vi "Puzzle 14-2.vi"() -> ()   [LabVIEW 2022 SP3]
panel:
  in  "delimited string":string="...#.O.#.#.O.O....#...O....#..#........OO.O#...O..O#O#.......O.O....O.....#...OO#.O....OOO..OO#..#..\n.##.....#.OOO.OO#...O.......O#..O.##OO.O.......O##....O....#O..O..#.#....#OO..#...O.O#.#...#....#O.O\nO...##.O.O.O.O..#.#.....#O....#..#O..O...O..OO..O...##.......OO#..OOO..#O..#.O#.O......#..#O..O..O.O\n..OO....OOO....O.O..OOO.....O........#...O.O.O.O..O#.O...O..#.#O........O.....#O...##....#...#.#....\n##.O.O#..O..##O.....O.#.....O.O#O.O..#...#...OO.##OOO...OO#...O...O........O.#.O.........#O.#...#.#.\n.#.O.O.....#..O###..O#.#..O....O.O....#...##.O..O.OOO..O.O..O#.O..O....#.#.O..#..##O...O....#O#.....\n.......O...##..O..O##..##...O....###.O.#.#.O......O...O.O......#O.....#..O..O#..##O.O#O##O....O#....\n.#O..#....##.##..O#..#..#..O........OO....#..##.O.#.O.O..OO.O.O#..#O##O......OO...O...OO...#....OO..\n#.....O#......O#.....#..O...#O..OO..OO.#O...O...O.........O...#O...O.....#.....#...#.....O##.O.....O\nOO.O..O...O......#.O......#O....#..#.#...O.O....O.#.O#...O........O......#.#O#.O...O.........#O....O\nO.O..O..#......O.O.OO...OO..##.....OO.....#.O...O.#.#...OO..OO.O.........#O..#.O...O#.#..O..OO.##O..\n..#.......O....#...#....##..O.O......O....O#.O..O..#.#.O#O.O.#...#.##.....O...O.O...O.#...O...O.#...\n.O...#..O.....O.O.....OO.O.O.......O..O..........#...O..O..O......O....#OOO...O#O...#.O#........O...\n.OO#....#.....O...#.###..#..O..O.....#O..#..OO...OOO#.O#..O#O........#..#.O..OOO#O#..O..OO........#.\n..O.....#..#..O.............#..O.O..O#.......#.O.........O.#..OO.O..#..##..O.O#O....OO.O.O.O.....O#.\n........#O..O#OO...#.##O.O....O...O..........##.#O..O......O..O.#...#O.O.OO...#.#OOO.#...O#....#.O.#\n.....O.O...#OO#.OO#......#..O.O..#.OO.......#...#.O.O#.O.#O.O#..#O##..OO...#......#.O....#.....O.#O.\n.O#OOOO...#.#..........O#.#.#.#.O....O..O...O...OOO.O.O.O..OO..O..O#.#...#....#...#O#.OO.O..#.O#....\nOO#OO..#.O.#....#..#.#..#O#.O#O#.#..O.O....#..O...OO..O..#........#.O...O#.#.....#....O.....#.O.....\n.O.....#...OO...#..O..#..O..O##..OO...O....#.O.#............###.O.#..O..O.........O..#.O..O.#OO.#...\n.##O.#.O.#....O..O..#..O.#.O..##O..O......OO...#...O..OO#....O..O#O.##.OO#...O#...#.......O.O#.#OO..\n.OO#O#...O..##.O......O..O.O....O...OOO.O..#...O#.#.O.OOO..#...#.##..OO..................OOOOO...###\n.#..##...####.O#...O........O...#O..O..O....O##O..O..OO..#.....#...O.....OO......OOO.#..O.##OO##...#\n....O#........O##.O...O#..#.O#O...O...O.O........#..#.#.O......O..#.....#.O..#.#..#..#O....O##...#..\n.O..OO.O##..O...O.OO....O.OOO..#O#.O##......O.O#....O#O.O......#.O..#O..#O.........#..OO....#.OO..O.\n.#OO..#OO.###........#...#..#.O..#O.O#O...O.#.....O...#......O.......#.O.#.##.O..#O.O###OOOO...#..O.\n##...OOO.#..........O#...O#.....OO...O#..OO.OO.#.OOO..OO....O..OOO...##O...O.........##O...#.#O.....\n.#....O.....#OO.O.OO..O......#.OO..#O...O..##O.#O....#O.OO..#O.OO...O..O.#..##...O......#O##OO.#.O..\n.#..O....O....#......#.O.##...OO.O.O...O.OO.O....#...#..O....O#O..#...#.#..#...OO......OOO...O..#...\n#.#OO.#....O.#.OO....#........O.O.##...O.#.................OOOO....O..#......O..#.#...O....#.O#OO.#O\n....O.O.......##..O.........OO#O..O.O#.#.#.O....#..OO.O..O#O....O..O.O......O.O.#..O.......O.O..O.O#\n...........#OO...O....#.O.#..#O.O#.....O..O.....O#.....OO.#O...#O.#O.#.....OO.O.O....OO......O#O.O..\nOOOO.OO..O....O.O...O..#.........O#.##OOO#.O..O.O.O......O..#..O..#..#.O..O....O#O.#OO..O.O...O#.##.\n##.O.#O.#OO#..........OO#.OO.#..#.#......#.OO...#.O.O.......O##....O..O..#.#.#O....O..##.#OO.O..O..O\n#O...OO..#.#....##.O#.#...##OO#........O#.O..O#.........O.O.#....O.#.O.......O..OOO......O#O.###.O..\n....O#....#..O...#.#.....O.O#O..#O....O...O.OO#...O..O#.##.O.....O...#..#.O.....O...O#..O.#...#.#O..\nO.OO......#..O...O.O....#...OO..O#.O..OO..#.##.....#....O.O#O#.O....O..#..OOO..O....O.O..#..O.O..O..\n.#..#..##O..O.....O#.#.O.O..O..OO..O.O..OO.##.O...O..O#........O.............#.OO..#......O..#O#OOO.\n.#..##...O.#..OO...O..#..#O#..#..##.O#.#.....#....O.O..O.........#.###...#.O##..O...#.O.OO..........\n........#O.......O...O#.#....#.O#....#..O.....OO........O...#.........##.....O...O#.O...O.O..#OO.O.#\n.#..#.O##..##.O#.#.......OO...OO#...#O#............#.#...#...O...#.O..#O.#.O.........O..OO.O...O.#..\n#.O#OO...OO.O.#...##........#....O.#.O.....##.#.O.O.O.#..O#...O..#......#..O...###O..OO..##..OO.#OOO\n.OO...#O....O##.O...O.#....O...#O.......O.....OO.O...O..#...OO.OO.O#...O##.....O..#.#...#OO......O..\n..O..#...O...##..O...O..OO.O.O.O.....#.....O.....O..#OOO.....OOOO#.#.O..O..#........O.#O#.#O..O.##..\n.....##.....O.....O#...##.OOO....O.O..O.#.#O........OO.....#...##...#.#......#....OO.O.....#O....#.#\n..O.OO#....O..O.#O.#OO#..#.O.##.#..#.OO##....O#...#..O.#..#...#.#....OOOO.#...OOOO..O.........##O.O.\nO.O.#......O#...O..#.......#O.O..OOOO..#....#.#.OO.O..#O......#.#....#...#..O....#O.OO..O.......#.#.\n...O.O....O#......#.O.O....O#.#..#O.#.....#...#...#.O#.........O.OO..O###...O....O.#.O.#.....##..O..\n.#.OO...O#O.....O#....O......OO...OO.OOOOOO##....#..#..#O.#.OO....O#..OO.#O........O#..O.O#.#.......\n#OO#.#.....O#OOO#...O.........#......O#.......O.....O#.#O...O........#....O...O.....#.......##.OOO#.\n..#.O##..#OO..#....#O....#....#..........#O...#...O.#.O.O###O..O..#...#.OO....##..O.O.O.....O..O....\n....OOO#.#......#..O.O......##O.#.O.#.O.OO....#..O.......#.....#O.O...##O###.##.##..#.O.#.O#..#..O#.\n......O#OO......#.#..#.O#OO#O..O#O.O##.......O...O........O......O#.....#..#....#...#.#..O...O##.#O.\n#..OO..O.O.....#O.O.#.#......O......O.#....O.#OO.........#.O.O#..#..#.O..O.#..#...#...O.#..........O\n..O#OOO#.#.....O.....O..##.#..OOO.O..#..O#...##O..OO...#....#..#...#...OO.....##OO#.OO...#.O....#.#.\n#.#O.............#....O#.....O.....O.##O.....#.#.#.....O....O...O...##..O...#........#O..##.#.....##\n.O.....O...#O.#.O#..O#........#.##...O##O..........O##.O......O..#....##....###......O##..##O..#.O#.\n.#...#..#..O.O.............#....O.OO.....OO#O.....OO..OOO#O.O.O.O...#...#.........OO..O#.O...#.##..#\n..O...#O#.......#OO..........OO#..#.....OO#...#OO.O#....OO....O..O..#....#OO......O#O...#......O..O.\nO.......O..O..#O.....O#O.........O##.O#.#.O.O....##....O.#....O....OOO..#O#...#...O.O#.O.....O.O#.O.\nO.#O....O..##....O.........##.OO###....O...O...O..O#O#...#O.O.O....#..O..#..#.O.......###..#....#..O\n.........O..#O...O..OO.....#...O..#O#.....O....#O#....##...#.OOOO.O..O#...O..O.O#.#..O.O..#..#.OO...\n...#.....#..OO.O.#.#.O.....O#...#..O...O..O..#...O..O.O..#...#.###..#..##O.#.#O.......O..##O.O.O#...\n.##O......O....#....O....#O..#.....#.O..O.O.O..#.#O.....O#.O...#.#O.#...#.........O....O....OO..O...\n.OO.O.O.O#O..O##.O...OO.....O..O....O....#..#...O.O...O....O.#.O......#O.#.O#O..O...O.O.#.O..O.#....\nO#..#.#..#..#...#.O...O.###.##.OO.O.#.OOO..O..#O.#.O...OO...O.OOO....#.....#OO.O##.O.#.#O...#.#.....\n.#.....#.........O.#.........#...OO..O.#.O...O##O...#..O.O.OO#....###.OO.....#..........#.#OO...O.O.\n........OO..O.O.#..O.#.......#.#O.OOO...OO.O............O#O#...O...#.O.....#...........O...#..OO.O#O\n..#.#.#...O....#O.......#...#...O###.O.....O.O.OO....#O...OO.O.O........O.O.#O.O....OO.....OO.....#.\n#..OOO#......O.#.O#...#..#..O..O.O.O.#...O#OOO.#...O.#.OO.#O..#....#..#O....O.#.O...O...O#OO...#....\n.....#.....##...O....#..O..O.....O#OO.#O#.....O...O.##.#........O..O........#.#......##......#..#..O\nO..O....O.##..#.#O##.#.....OO....O.##O......#...#..OO.O.....#...#........O..O#O##.O.......#..##O..##\n#.....#O....O...#OOO#..O#.O.....O..OO.#..#.#.O#..O..O#.O###....O......O.#.O..#O.....#.......##O.O..O\nO.O.#..#....O....O.......#.O..O#O#.O..........#O.....#OO.O...#.OO.....#...O....OO....#...O....O.#..O\n..#...OO....OO......O....#..#..........##..##..#.....##...#..#O.....#OO......#........O.....O..O...#\n.OO#...O#.O....#.........OO#...O#..O.#..O.O.O.#O......##.O.......O...O...###.O......O....O...#.OO#..\n..O..O#O.#..O.#O...OOO#O.#.O....O.#......O....#....###....OO......O...#...OO.#....O........O#..#..OO\n#..OO..O......#...##..O#.O........O.O...##.#O...O...#O#.O.O....#.............#.O#.#..O..#..OO#.....#\n#..........O...O##.O#..O..OO..O.....#O.#.O......#......O.O....##.O#OO..O.O..O.O.O..#..O....O..#....O\n.O.O...O.#..O.O....#.#.O.O.##.##..O..#OOOO.###...#O...#...O.....O...#.##.OO..O.#..#.O.#.......O....#\n#....#....OOOOOOO.#...OO....##O.#..#......O..#..........O......##..O..###..#.O....O.......OO......#.\n.O.O..##.O.#O.#...#....O..O.....#..##......O.......O..O#.O##.#........O..#.O.#.O.O..##..###..##.#...\n..OOO..O##..OOOO.O.....OO##..O..O.#....#.....OO......O.OOO#...#O.OO...O.O......O#..O.##....###...#.O\n....O...O.O....#..O#.O.....O.O.#.......O##...O#..OO.O.O##...#.....O#.###....O....#O.........OO..O.O.\nO#.O......##..#.#..............#......#.#.OO#......##O#OO..OOO..##.O##....#..O...#......##O.O##...OO\n...#OO....OO...O#.#..##....OO.#..#O......O#....#.O.....O.#O..OO.#..OO...O#.O#....O.#.OO.O.O#..O.....\n#..O.OO#O...O..O..........#..#.#..#..#O.....#O#..O....#..O...O.#.#O#.#OO.....OOO.#..#.........O...O#\n....O......#..........O...#.....OOOO........#.#OO.O............O...#....O........#....#....#........\n...O.......###...O.O...#O.##O.OOO.........O.###.O.......O....O.O...O.#.....#..#O..#..OO..O.O...O....\nO.O#....##.O.O.....O....#............OO.#O...O..#...##.#.#O#O.#.....O......O....#.OO#.O#....#.....O.\n..O####.O.........O...........OO..OO.#.....O.......#..O#.O....O#...##.......#.#....O..O..O#..##.....\n.#..#......O.##.O.OOO.O.OO....O.......#......#.O...OOOO...O..#..#.O.#......O...O#.#.O.#.O....O....O.\n##....O.O..O..O.#...O##.......O....#...#OOO.O..##.....#....O.......#O..#.#O..O.#.......O..#.O.O#.O##\n...O....O#O.#...#......#..O.O.O.O...O.....O..O.#..#.....O#...OO...#.O.O....#..OOO...#.....OO.OO..O..\nO##.O.##.O#OO...OO...OO..O....OO#O.#O..O.O....OO..........O..#.O.#O#.......O.O..#O#....#..#...#O..#.\n.#.#..........#.......#..OO#....O.#.#.O.....OO.#.O..#.#.O....#..O....#..#..O.#O#O.....#.O.O.#O.O.#O.\n.O.#....##O...#..OOO.#......#...#.O.......OO....#.......#..#.OOO........OO..O..###O##..O.....O##....\nOO##..O#....O.##.......O...#........O.O...#O#.#.OOO....#......#.#O.O.O..O..O...#.#.O.O.OOO.O#O......\n#O...#....OOO.O...#O....O...O..........O..#..O#.O..#O.....#......#.#..#.OO..#....#O#....O...O....##.\n.OOOO......##.#O.#O...#......O..#..O..#.O...O.OO...............#O...O..##..#.#....O...O..O.##..O.O.."
  in  "Numeric":i32=1000000000
  out "sum":i32
  out "unsigned byte array 2":u8[][](array[numeric])
  out "unsigned byte array":u8[][](array[numeric])
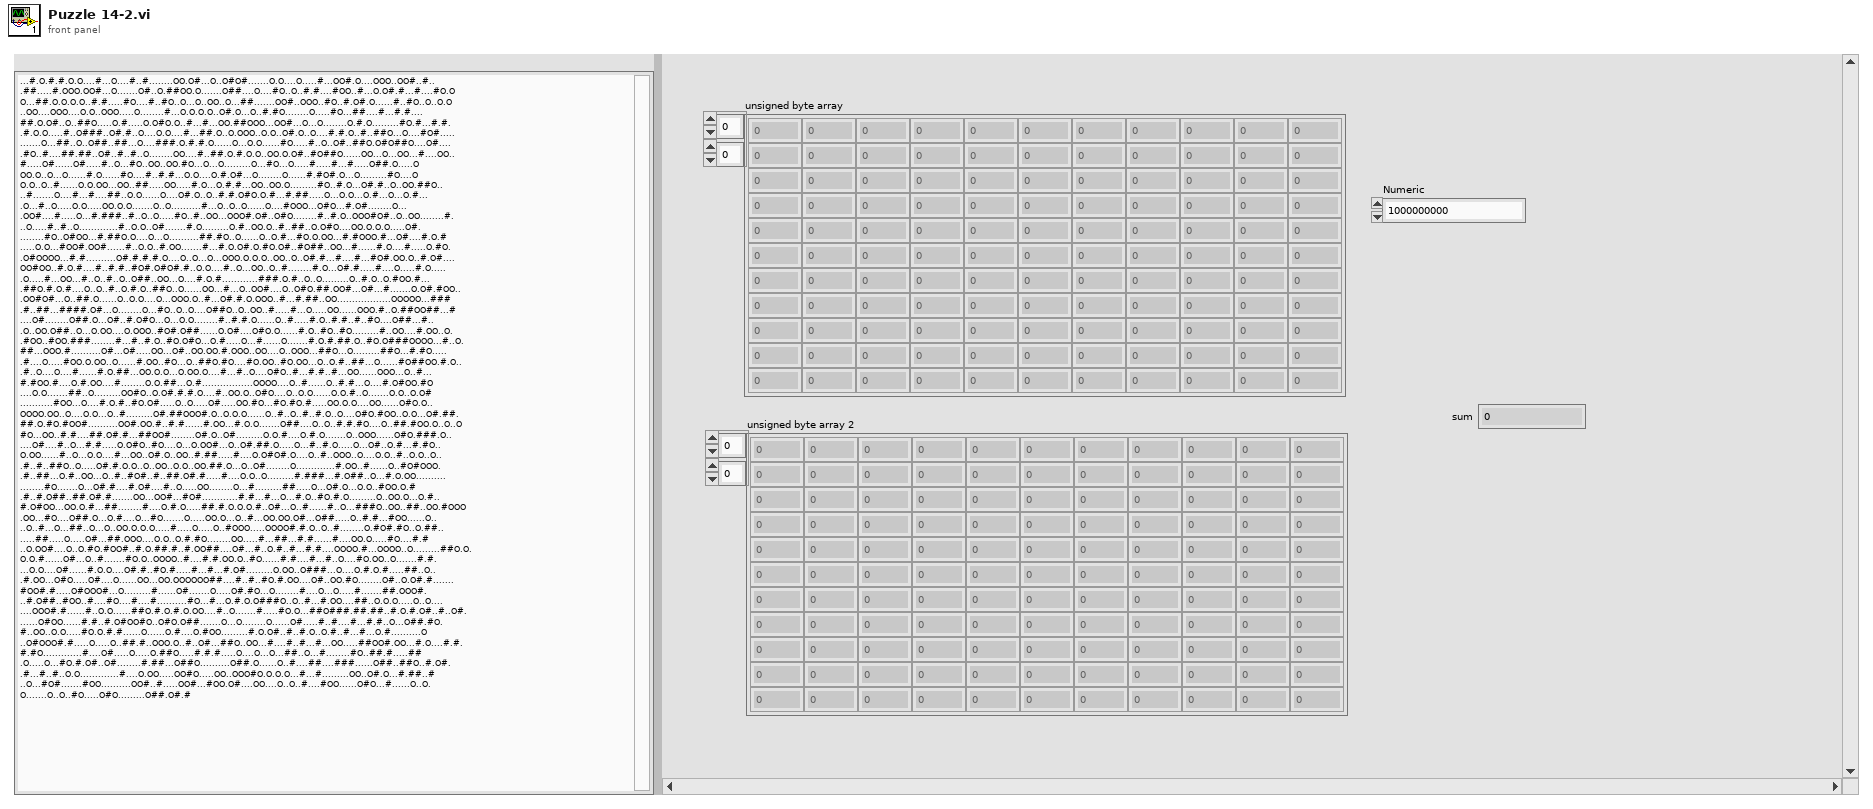
[diagram p1: front panel]
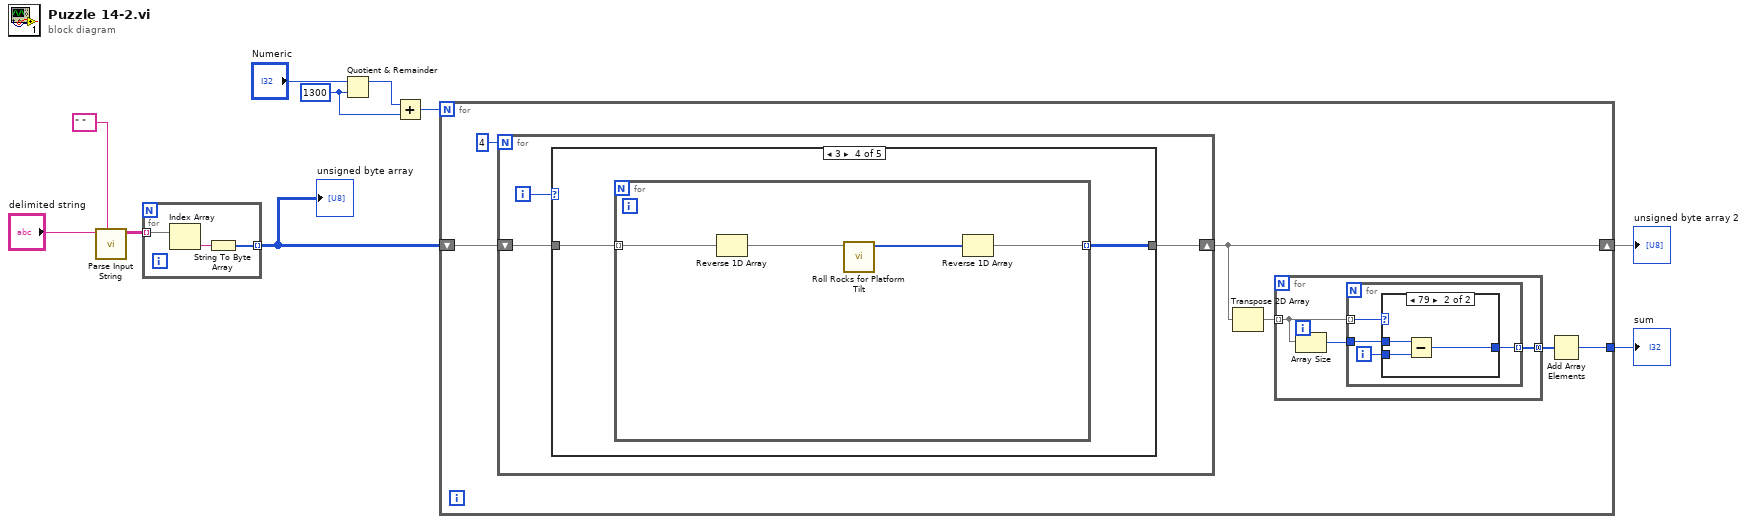
[diagram p0: block diagram]
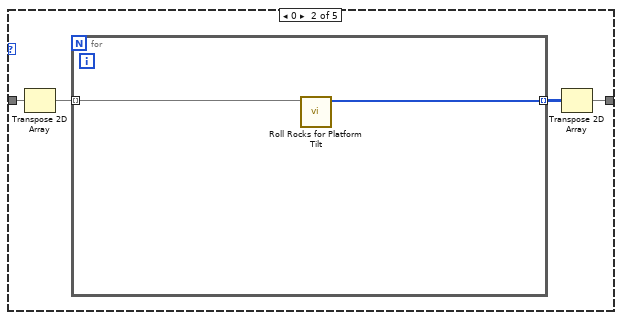
[diagram p4: hidden frame]
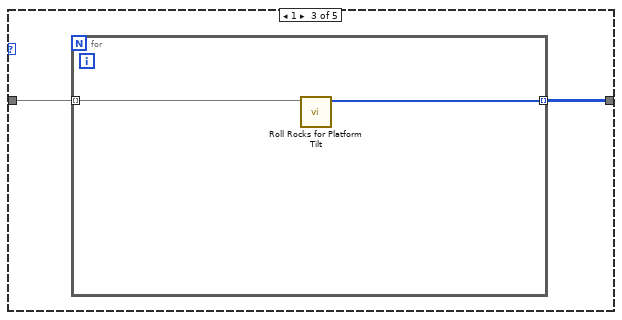
[diagram p5: hidden frame]
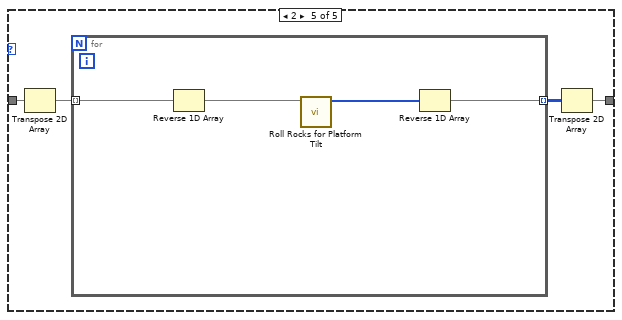
[diagram p6: hidden frame]
diagram:
  w3 = 1300 ("y")
  n1 = call "Parse Input String.vi"("delimiter (Tab)"=" ", "delimited string"="delimited string") -> ("parsed string"=w8:string[][])  [unwired: 9 in]
  n2 = for {
    tunnel: w8 -> [w13] mode=indexing
    tunnel: [w11] -> w7 mode=indexing
    n3 = Index Array(array=w13) -> (element=w12:string)  [unwired: 1 in]
    n4 = String To Byte Array(string=w12) -> (unsigned byte array=w11:u8[])
  }
  "unsigned byte array" <- w7
  n5 = Quotient & Remainder(x="Numeric", y=w3) -> (x-y*floor(x/y)=w2:i32)  [unwired: 1 out]
  n6 = Add(x=w2, y=w3) -> (x+y=w1:i32)
  n7 = for {
    N: w1 -> [_]
    shift-right: [w14] -> w6
    shift-left: w7 -> [w19]
    tunnel: [w15] -> w5
    n8 = for {
      N: 4 -> [_]
      shift-right: [w31] -> w14
      shift-left: w19 -> [w32]
      i -> [w30]
      n9 = case shown="3" w30 {
        tunnel: w32 -> [w33 w37 w41 w45 w53]
        tunnel: [w33 w34 w40 w44 w50] -> w31
        frame Default {
        }
        frame 0 {
          n10 = Transpose 2D Array(2D array=w37) -> (transposed array=w36:u8[][])
          n11 = for {
            tunnel: w36 -> [w39] mode=indexing
            tunnel: [w38] -> w35 mode=indexing
            n12 = call "Roll Rocks for Platform Tilt.vi"("Array in"=w39) -> ("Array out"=w38:u8[])  [unwired: 10 in]
          }
          n13 = Transpose 2D Array(2D array=w35) -> (transposed array=w34:u8[][])
        }
        frame 1 {
          n14 = for {
            tunnel: w41 -> [w43] mode=indexing
            tunnel: [w42] -> w40 mode=indexing
            n15 = call "Roll Rocks for Platform Tilt.vi"("Array in"=w43) -> ("Array out"=w42:u8[])  [unwired: 10 in]
          }
        }
        frame 3 {
          n16 = for {
            tunnel: w45 -> [w49] mode=indexing
            tunnel: [w46] -> w44 mode=indexing
            n17 = Reverse 1D Array(array=w49) -> (reversed array=w47:u8[])
            n18 = call "Roll Rocks for Platform Tilt.vi"("Array in"=w47) -> ("Array out"=w48:u8[])  [unwired: 10 in]
            n19 = Reverse 1D Array(array=w48) -> (reversed array=w46:u8[])
          }
        }
        frame 2 {
          n20 = Transpose 2D Array(2D array=w53) -> (transposed array=w52:u8[][])
          n21 = for {
            tunnel: w52 -> [w57] mode=indexing
            tunnel: [w54] -> w51 mode=indexing
            n22 = Reverse 1D Array(array=w57) -> (reversed array=w55:u8[])
            n23 = call "Roll Rocks for Platform Tilt.vi"("Array in"=w55) -> ("Array out"=w56:u8[])  [unwired: 10 in]
            n24 = Reverse 1D Array(array=w56) -> (reversed array=w54:u8[])
          }
          n25 = Transpose 2D Array(2D array=w51) -> (transposed array=w50:u8[][])
        }
      }
    }
    n26 = Transpose 2D Array(2D array=w14) -> (transposed array=w17:u8[][])
    n27 = for {
      tunnel: w17 -> [w22] mode=indexing
      tunnel: [w20] -> w16 mode=concatenating
      n28 = Array Size(array=w22) -> (size(s)=w21:i32)
      n29 = for {
        tunnel: w22 -> [w26] mode=indexing
        tunnel: w21 -> [w25]
        tunnel: [w23] -> w20 mode=indexing
        i -> [w24]
        n30 = case shown="79" w26 {
          tunnel: w25 -> [_ w29]
          tunnel: w24 -> [_ w28]
          tunnel: [_ w27] -> w23
          frame Default {
          }
          frame 79 {
            n31 = Subtract(x=w29, y=w28) -> (x-y=w27:i32)
          }
        }
      }
    }
    n32 = Add Array Elements(numeric array=w16) -> (sum=w15:i32)
  }
  "unsigned byte array 2" <- w6
  "sum" <- w5
